vi "Configure Digital Input.vi"(0 "VISA resource name":refnum<visa-resource-name>, 1 "Unit Address (1)":i16=1, 2 "Name (DIGIT IN1)":string="DIGIT IN1", 5 "Digital Input (1)":i16=1, 7 "Function (0: Off)":u16(ring) items=["Off", "Panel Lock", "Reset Alarm", "Control Outputs Off", "All Outputs Off", "Digital Outputs Off", "Start Profile", "Pause Profile", "Resume Profile", "Terminate Profile", "Wait For Event"], 9 "Condition (0: Low)":u16(ring) items=["Low", "High"], 11 "error in (no error)":errorcluster {"code" format="%.0x"}) -> (4 "VISA resource name out":refnum<visa-resource-name>, 15 "error out":errorcluster {"code" format="%.0x"})   [LabVIEW 2010]
doc: "This VI configures digital inputs."
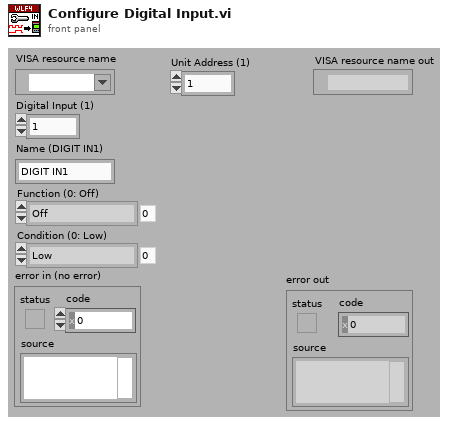
[diagram p1: front panel]
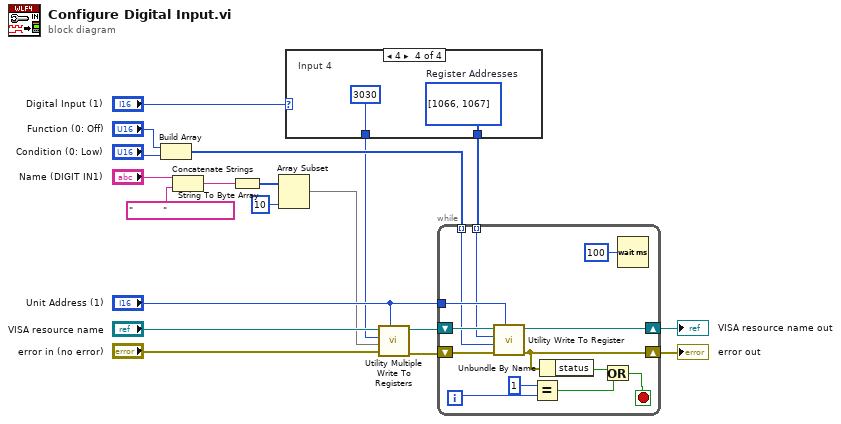
[diagram p0: block diagram]
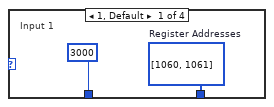
[diagram p2: hidden frame]
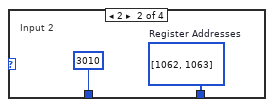
[diagram p3: hidden frame]
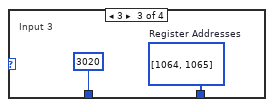
[diagram p4: hidden frame]
diagram:
  n1 = Build Array("Function (0: Off)", "Condition (0: Low)") -> (w17:u16[])
  n2 = Concatenate Strings("Name (DIGIT IN1)", "          " ("string")) -> (w3:string)
  n3 = String To Byte Array(string=w3) -> (unsigned byte array=w5:u8[])
  n4 = Array Subset(array=w5, length=10) -> (w2:u8[])  [unwired: 1 in]
  n5 = case shown="4" "Digital Input (1)" {
    tunnel: [w21 w23 w25 w27] -> w13
    tunnel: [3000 3010 3020 3030] -> w7
    frame 1, Default {
      w21 = i32[] [1060, 1061]  # Register Addresses
      # "Input 1"
    }
    frame 2 {
      w23 = i32[] [1062, 1063]  # Register Addresses
      # "Input 2"
    }
    frame 3 {
      w25 = i32[] [1064, 1065]  # Register Addresses
      # "Input 3"
    }
    frame 4 {
      w27 = i32[] [1066, 1067]  # Register Addresses
      # "Input 4"
    }
  }
  n6 = call "Utility Multiple Write To Registers.vi"("Unit Address (1)"="Unit Address (1)", "error in (no error)"="error in (no error)", "Array Of Data"=w2, "Register Address (0)"=w7, "VISA resource name"="VISA resource name") -> ("error out"=w11:errorcluster, "VISA resource name out"=w9:refnum<visa-resource-name>)  [unwired: 5 in]
  n7 = while {
    tunnel: "Unit Address (1)" -> [w40]
    shift-right: [w37] -> w19
    shift-left: w9 -> [w39]
    shift-right: [w33] -> w18
    shift-left: w11 -> [w38]
    tunnel: w13 -> [w35] mode=indexing
    tunnel: w17 -> [w34] mode=indexing
    i -> [w30]
    stop <- w32 stop-if-true
    n8 = call "Utility Write To Register.vi"("Unit Address (1)"=w40, "error in (no error)"=w38, "Data (0)"=w34, "Register Address (0)"=w35, "VISA resource name"=w39) -> ("error out"=w33:errorcluster, "VISA resource name out"=w37:refnum<visa-resource-name>)  [unwired: 5 in]
    n9 = Equal?(x=1, y=w30) -> (x = y?=w29:bool)
    n10 = Unbundle By Name(w33) -> ("status"=w31:bool)
    n11 = Or(x=w31, y=w29) -> (x .or. y?=w32:bool)
    n12 = Wait (ms)(milliseconds to wait=u32 100) -> ()  [unwired: 1 out]
  }
  "error out" <- w18
  "VISA resource name out" <- w19
